vi "GYRO_Read_Plot.vi"(0 "I2C Ref Out":T1, 5 "PmodGYRO address":u8, 7 "reset integrator":bool, 11 "error in (no error)":errorcluster) -> (1 "X rate":dbl format="%.2f", 2 "Y rate":dbl format="%.2f", 3 "integral x(t)":dbl, 4 "DATA 2":u8[](array[numeric]) format="%02x", 6 "integral x(t) 3":dbl, 8 "Numeric":dbl format="%.2f", 10 "integral x(t) 2":dbl, 12 "Numeric 2":dbl format="%.2f", 13 "Numeric 3":dbl format="%.2f", 14 "Z rate":dbl format="%.2f", 15 "error out":errorcluster)   [LabVIEW 2021]
uses:
  <vilib>/myRIO/Instrument Drivers/Onboard IO/I2C/typedefs/I2C Reference.ctl
  <vilib>/myRIO/Common/Instrument Driver Framework/Utilities/typedefs/myRIO Generic Hardware Reference.ctl
  <vilib>/myRIO/Common/Instrument Driver Framework/Utilities/typedefs/Hardware Version Enum.ctl
  <vilib>/myRIO/Common/Instrument Driver Framework/Utilities/typedefs/myRIO v1.0 Reference.ctl
  <vilib>/myRIO/Common/Instrument Driver Framework/Utilities/typedefs/Generic FPGA Reference.ctl
  <vilib>/myRIO/Common/Instrument Driver Framework/myRIO v1.0/I2C/typedefs/I2C Channels Enum.ctl
  <vilib>/myRIO/Instrument Drivers/Onboard IO/I2C/typedefs/I2C Configuration.ctl
  <vilib>/myRIO/Instrument Drivers/Onboard IO/I2C/typedefs/I2C Transfer Rate.ctl
  <vilib>/Utility/error.llb/Error Cluster From Error Code.vi
  <vilib>/myRIO/Common/Instrument Driver Framework/myRIO v1.0/I2C/vis/myRIO v1.0 Write I2C.vi
  <vilib>/myRIO/Common/Instrument Driver Framework/myRIO v1.0/I2C/vis/myRIO v1.0 Read I2C.vi
  <vilib>/myRIO/Instrument Drivers/Onboard IO/I2C/I2C.lvlib
  <vilib>/ptbypt/NI_PtbyPt.lvlib
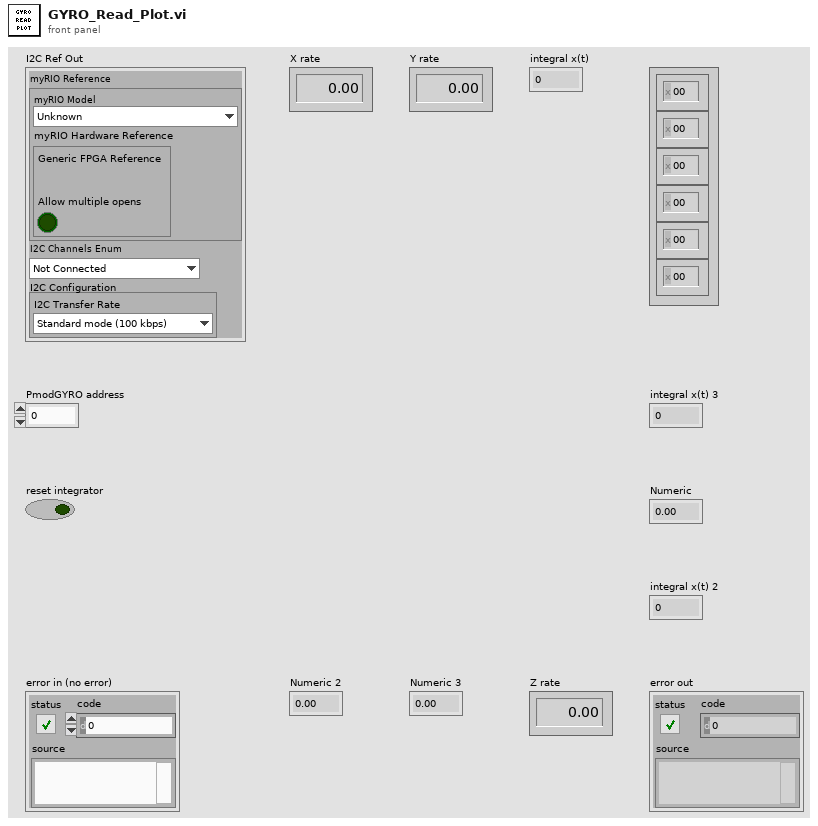
[diagram p1: front panel]
types:
  T1 = typedef "I2C.lvlib/I2C Reference.ctl" = cluster{"myRIO Reference":T2, "I2C Channels Enum":T6, "I2C Configuration":T7}
  T2 = typedef "myRIO Generic Hardware Reference.ctl" = cluster{"myRIO Model":T3, "myRIO Hardware Reference":T4}
  T3 = typedef "Hardware Version Enum.ctl" = enum16{"Unknown", "myRIO-1900", "myRIO-1950", "roboRIO", "NI ELVIS RIO CM", "ELVIS III"}
  T4 = typedef "myRIO v1.0 Reference.ctl" = cluster{"Generic FPGA Reference":T5, "Allow multiple opens":bool}
  T5 = typedef "Generic FPGA Reference.ctl" = refnum<k20>
  T6 = typedef "I2C Channels Enum.ctl" = enum16{"Not Connected", "A/I2C", "B/I2C", "I2C/I2C"}
  T7 = typedef "I2C.lvlib/I2C Configuration.ctl" = cluster{"I2C Transfer Rate":T8}
  T8 = typedef "I2C.lvlib/I2C Transfer Rate.ctl" = enum16{"Standard mode (100 kbps)", "Fast mode (400 kbps)"}
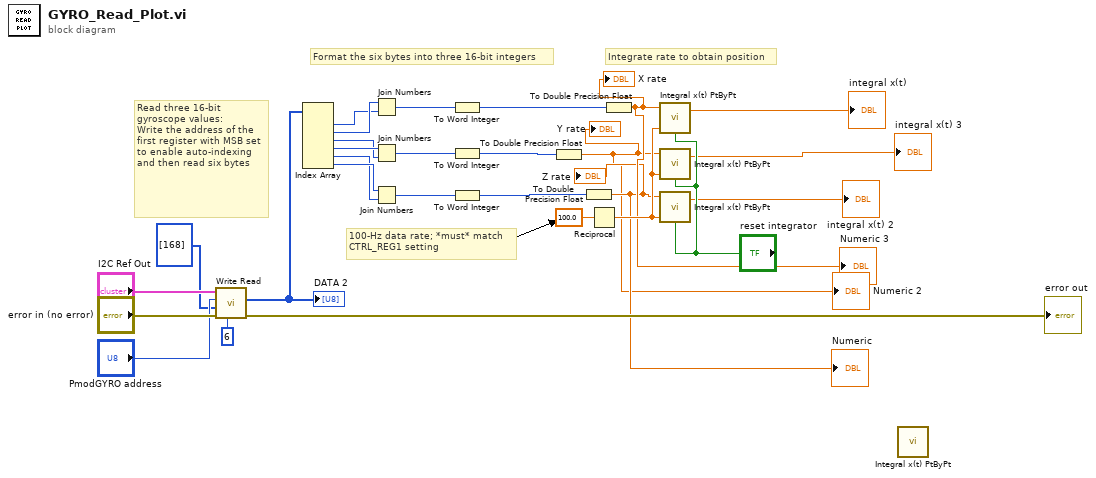
[diagram p0: block diagram]
diagram:
  # "100-Hz data rate; *must* match\nCTRL_REG1 setting"
  # "Integrate rate to obtain position"
  # "Read three 16-bit gyroscope values:\nWrite the address of the first register with MSB set to enable auto-indexing and then read six bytes"
  # "Format the six bytes into three 16-bit integers"
  n1 = call <vilib>:"Write Read.vi"("Byte Count"=u32 6, "error in (no error)"="error in (no error)", "Bytes to Write"=u8[] [168], "Slave Address (7-bit)"="PmodGYRO address", "I2C Ref In"="I2C Ref Out") -> ("error out"=→"error out":errorcluster, "Bytes Read"=w19:u8[])  [unwired: 3 in, 1 out]
  "DATA 2" <- w19
  n2 = Index Array "Index Array"(array=w19) -> (element #1=w9:u8, element #2=w10:u8, element #3=w11:u8, element #4=w12:u8, element #5=w13:u8, element #6=w14:u8)  [unwired: 6 in]
  n3 = Join Numbers(hi=w10, lo=w9) -> ((hi.lo)=w6:u16)
  n4 = Join Numbers(hi=w12, lo=w11) -> ((hi.lo)=w7:u16)
  n5 = Join Numbers(hi=w14, lo=w13) -> ((hi.lo)=w8:u16)
  n6 = To Word Integer(number=w6) -> (16bit integer=w20:i16)
  n7 = To Word Integer(number=w7) -> (16bit integer=w3:i16)
  n8 = To Word Integer(number=w8) -> (16bit integer=w21:i16)
  n9 = To Double Precision Float(number=w3) -> (double precision float=w2:dbl)
  "Y rate" <- w2
  "Numeric 2" <- w2
  n10 = To Double Precision Float(number=w21) -> (double precision float=w4:dbl)
  "Z rate" <- w4
  "Numeric" <- w4
  n11 = Reciprocal(x=100.0 ("dt")) -> (1/x=w25:dbl)
  n12 = To Double Precision Float(number=w20) -> (double precision float=w5:dbl)
  "X rate" <- w5
  "Numeric 3" <- w5
  n13 = call <vilib>:"Integral x(t) PtByPt.vi"("initialize"="reset integrator", "dt"=w25, "x"=w5) -> ("integral x(t)"=→"integral x(t)":dbl)  [unwired: 1 in, 1 out]
  n14 = call <vilib>:"Integral x(t) PtByPt.vi"("initialize"="reset integrator", "dt"=w25, "x"=w2) -> ("integral x(t)"=→"integral x(t) 3":dbl)  [unwired: 1 in, 1 out]
  n15 = call <vilib>:"Integral x(t) PtByPt.vi"("initialize"="reset integrator", "dt"=w25, "x"=w4) -> ("integral x(t)"=→"integral x(t) 2":dbl)  [unwired: 1 in, 1 out]
  n16 = call <vilib>:"Integral x(t) PtByPt.vi"() -> ()  [unwired: 4 in, 2 out]
